vi "CRC.vi"() -> ()   [LabVIEW 2019]
panel:
  out "CRC =   2":u16 format="%x"
  in  "DATA PACKET":string
  out "CRC =":u16 format="%x"
  # "Polynom X16+X12+X5+1"
  # "Felica and 14443 Type A - GOOD"
  # "15693 and 14443 Type B"
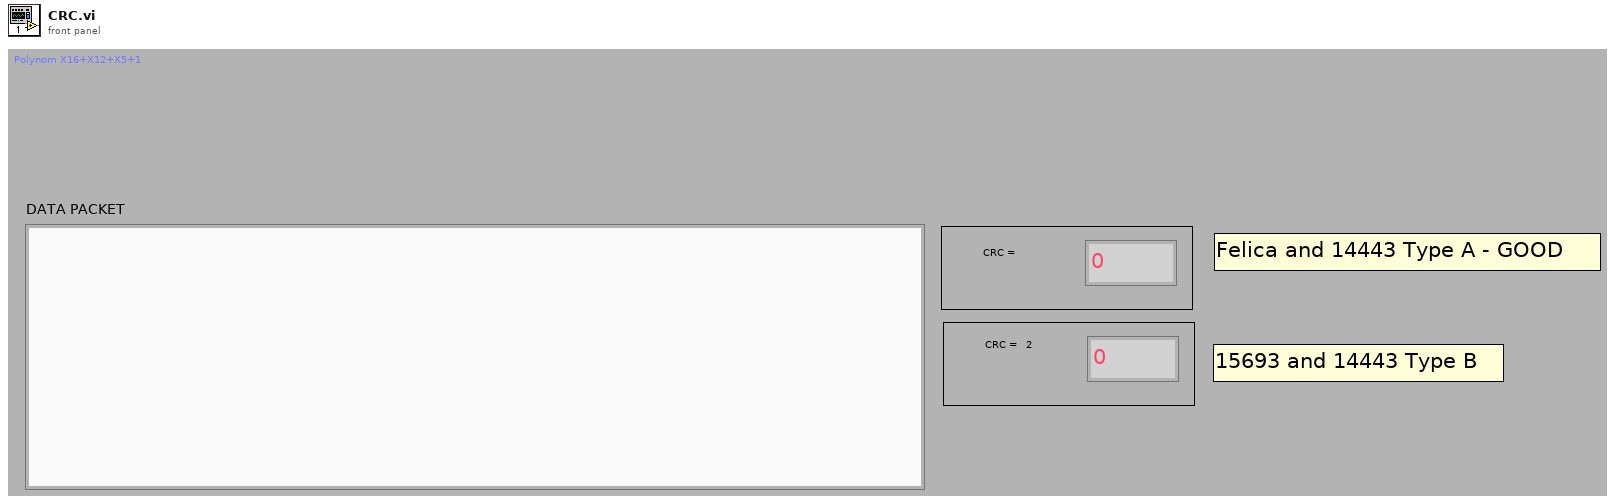
[diagram p1: front panel]
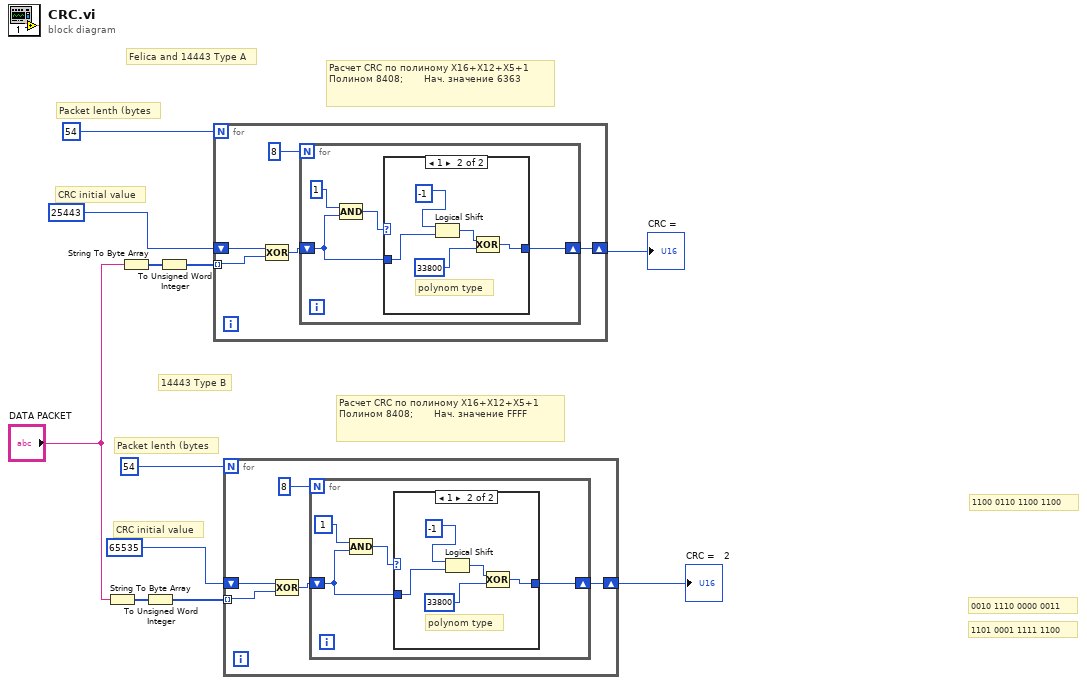
[diagram p0: block diagram]
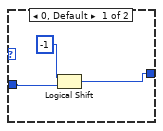
[diagram p2: hidden frame]
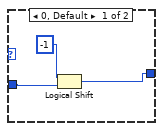
[diagram p3: hidden frame]
diagram:
  # "Felica and 14443 Type A"
  # "Packet lenth (bytes"
  # "CRC initial value"
  # "Расчет CRC по полиному X16+X12+X5+1\nПолином 8408;       Нач. значение 6363"
  # "1101 0001 1111 1100"
  # "0010 1110 0000 0011"
  # "1100 0110 1100 1100"
  # "14443 Type B"
  # "Packet lenth (bytes"
  # "CRC initial value"
  # "Расчет CRC по полиному X16+X12+X5+1\nПолином 8408;       Нач. значение FFFF"
  n1 = String To Byte Array(string="DATA PACKET") -> (unsigned byte array=w11:u8[])
  n2 = String To Byte Array(string="DATA PACKET") -> (unsigned byte array=w5:u8[])
  n3 = To Unsigned Word Integer(number=w11) -> (unsigned 16bit integer=w2:u16[])
  n4 = To Unsigned Word Integer(number=w5) -> (unsigned 16bit integer=w4:u16[])
  n5 = for {
    N: 54 -> [_]
    shift-right: [w13] -> w3
    shift-left: u16 25443 -> [w14]
    tunnel: w4 -> [w12] mode=indexing
    n6 = Compound Arithmetic op=XOR(w14, w12) -> (w15:u32)
    n7 = for {
      N: 8 -> [_]
      shift-right: [w19] -> w13
      shift-left: w15 -> [w18]
      n8 = Compound Arithmetic op=AND(u16 1, w18) -> (w17:u32)
      n9 = case shown="1" w17 {
        tunnel: [w22 w27] -> w19
        tunnel: w18 -> [w21 w24]
        frame 0, Default {
          n10 = Logical Shift(y=i16 -1, x=w21) -> (x << y=w22:u32)
        }
        frame 1 {
          # "polynom type"
          n11 = Logical Shift(y=i16 -1, x=w24) -> (x << y=w26:u32)
          n12 = Compound Arithmetic op=XOR(w26, u32 33800) -> (w27:u32)
        }
      }
    }
  }
  "CRC =" <- w3
  n13 = for {
    N: 54 -> [_]
    shift-right: [w30] -> w1
    shift-left: u16 65535 -> [w31]
    tunnel: w2 -> [w29] mode=indexing
    n14 = Compound Arithmetic op=XOR(w31, w29) -> (w32:u32)
    n15 = for {
      N: 8 -> [_]
      shift-right: [w36] -> w30
      shift-left: w32 -> [w35]
      n16 = Compound Arithmetic op=AND(u16 1, w35) -> (w34:u32)
      n17 = case shown="1" w34 {
        tunnel: [w39 w44] -> w36
        tunnel: w35 -> [w38 w41]
        frame 0, Default {
          n18 = Logical Shift(y=i16 -1, x=w38) -> (x << y=w39:u32)
        }
        frame 1 {
          # "polynom type"
          n19 = Logical Shift(y=i16 -1, x=w41) -> (x << y=w43:u32)
          n20 = Compound Arithmetic op=XOR(w43, u32 33800) -> (w44:u32)
        }
      }
    }
  }
  "CRC =   2" <- w1
